vi "CTB4.vi"() -> ()   [LabVIEW 2015]
uses:
  <vilib>/Instr/_visa.llb/VISA Configure Serial Port (Instr).vi
  <vilib>/Utility/file.llb/Write Delimited Spreadsheet (I64).vi
panel:
  out "Mixed Signal Graph 2":T1(graph)
  in  "tiempo de muestreo":u32
  in  "timeout (10sec)":u32=10000
  in  "stop bits (10: 1 bit)":u16(ring)=10 items=["1.0"=10, "1.5"=15, "2.0"=20]
  in  "data bits (8)":u16=8 min=5 max=8 step=1
  in  "baud rate (9600)":u32=9600
  in  "VISA resource name 2":refnum<visa-resource-name>
  in  "Archivo":path
  out "?":u32[][](array[numeric])
  out "Muestras":i32
  in  "?":bool
  out "read buffer":string
  # "CH2"
  # "CH3"
  # "CH4"
  # "CH5"
  # "CH7"
  # "CH1"
  # "CH6"
  # "CH8"
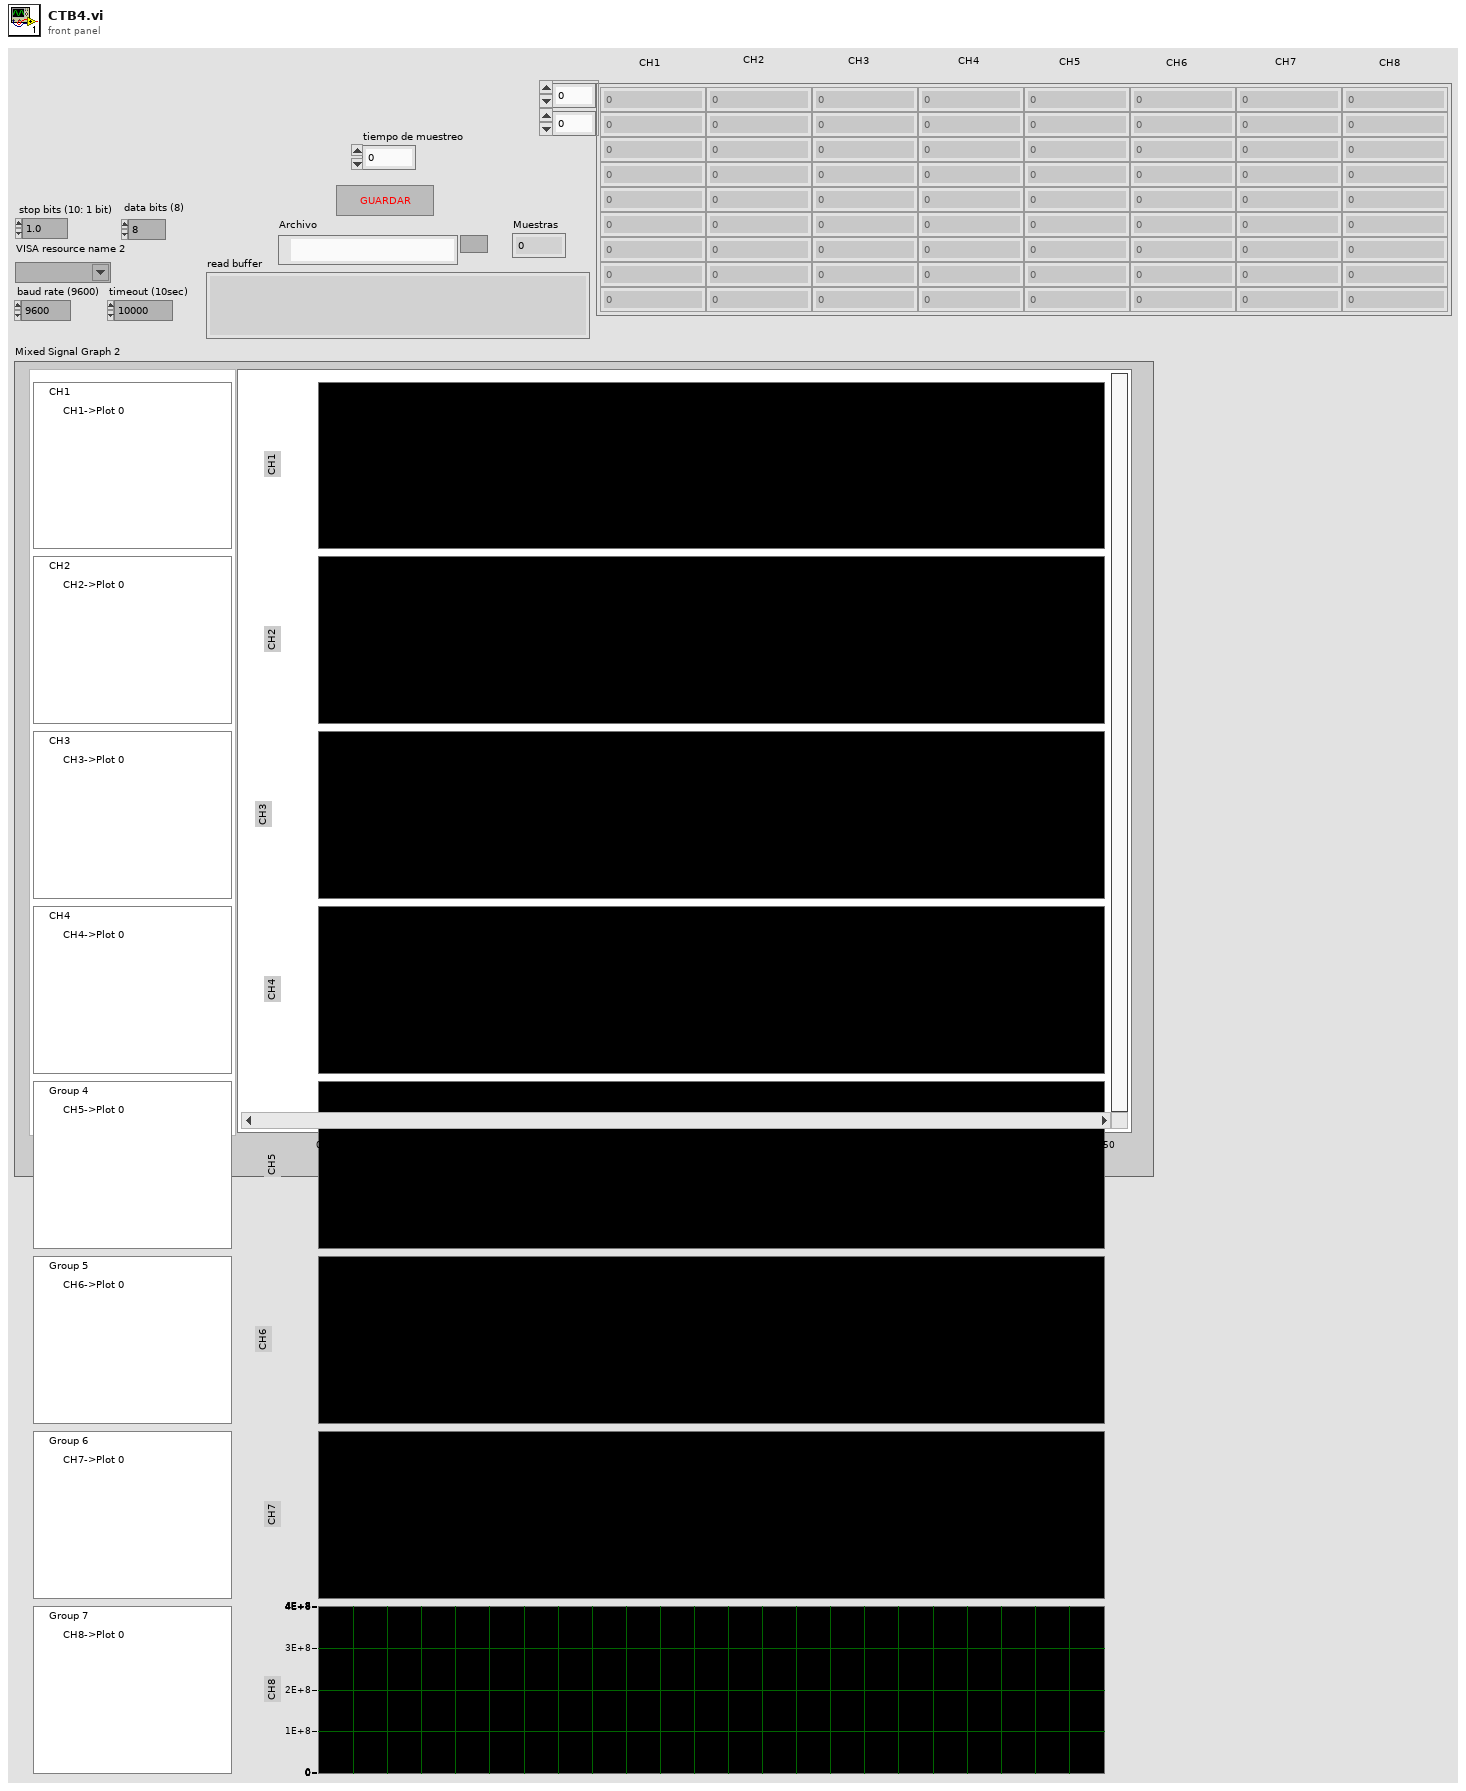
[diagram p1: front panel]
types:
  T1 = cluster{i32[], i32[], i32[], i32[], i32[], i32[], i32[], i32[]}
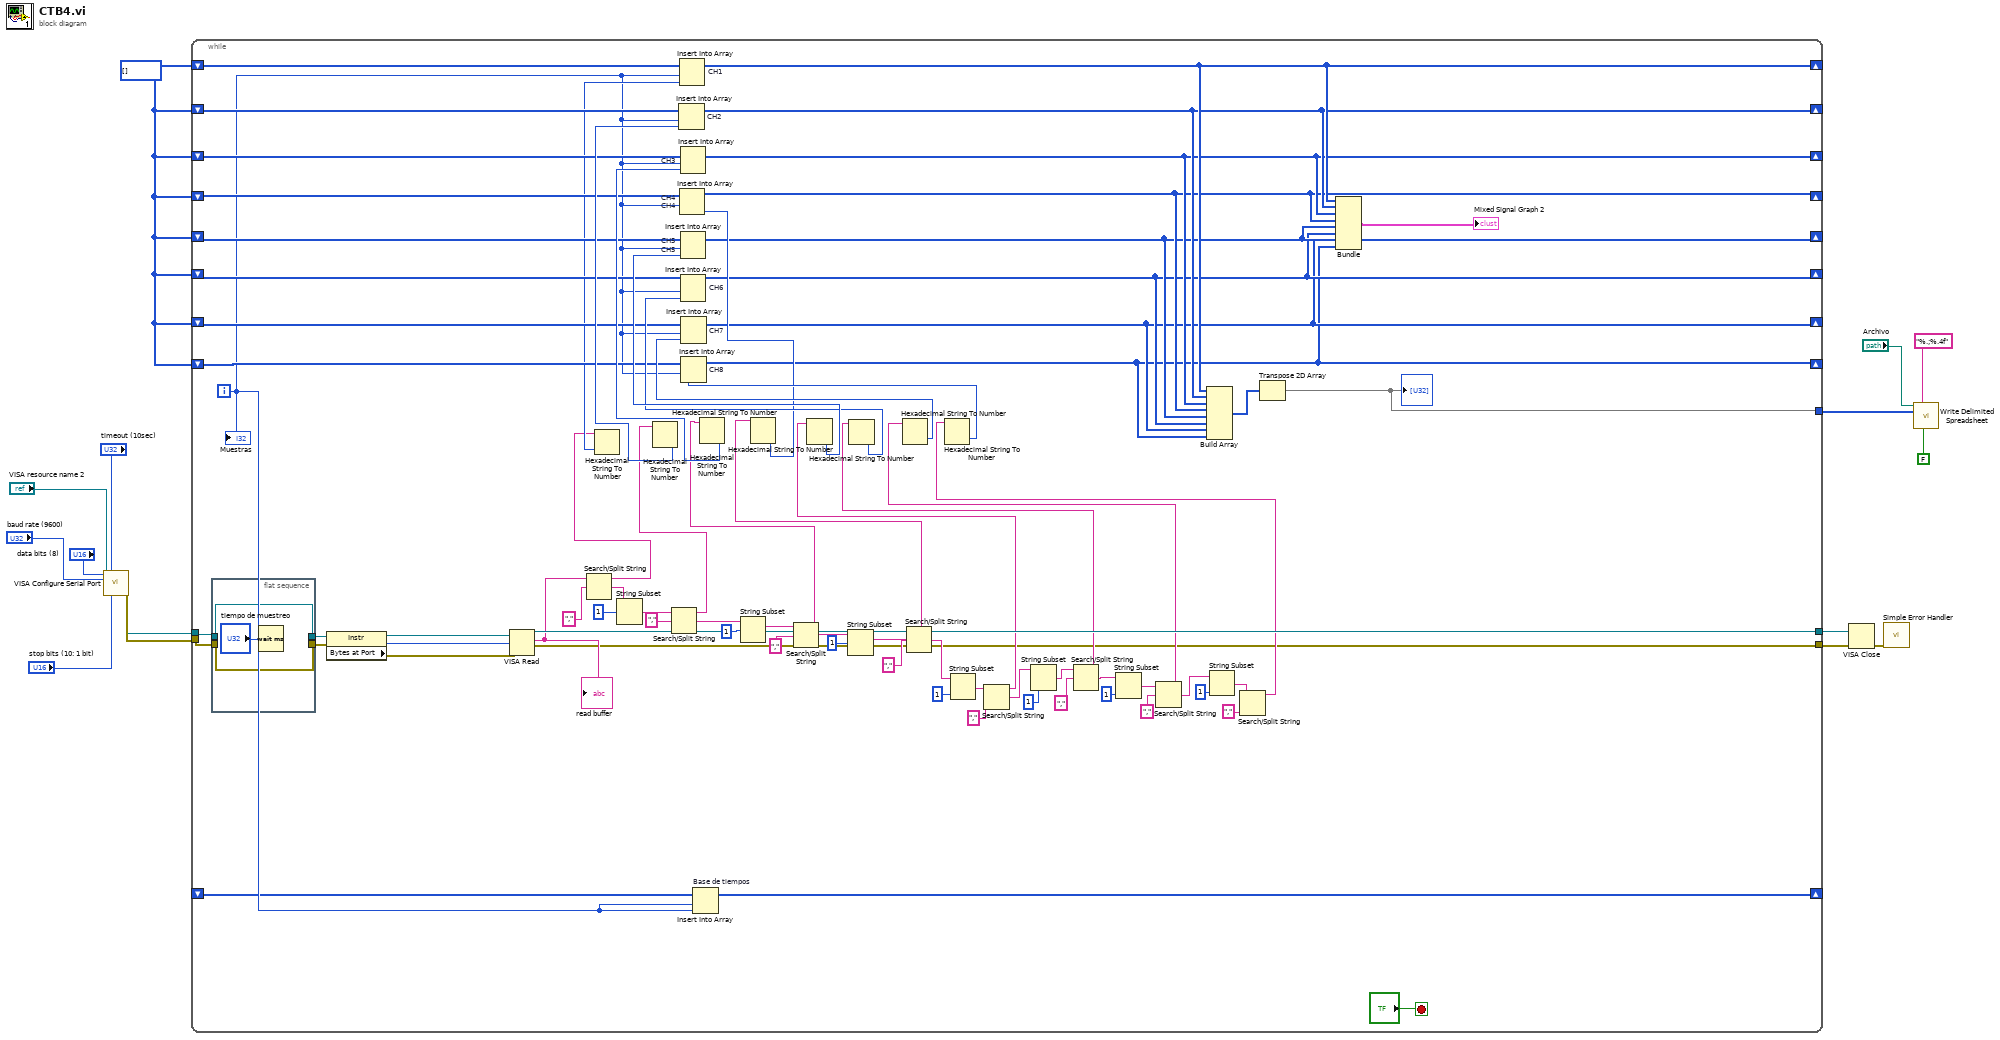
[diagram p0: block diagram]
diagram:
  w2 = i32[] []
  n1 = call-poly "VISA Configure Serial Port"("VISA resource name"="VISA resource name 2", "timeout (10sec)"="timeout (10sec)", "baud rate (9600)"="baud rate (9600)", "data bits (8)"="data bits (8)", "stop bits (10: 1 bit)"="stop bits (10: 1 bit)") -> ("VISA resource name out"=w5:refnum<visa-resource-name>, "error out"=w6:errorcluster)  [unwired: 9 in]
  n2 = while {
    shift-right: [w24] -> _
    shift-left: w2 -> [w33]
    shift-right: [w23] -> _
    shift-left: w2 -> [w86]
    shift-right: [w22] -> _
    shift-left: w2 -> [w83]
    shift-right: [w21] -> _
    shift-left: w2 -> [w78]
    shift-right: [w20] -> _
    shift-left: w2 -> [w77]
    shift-right: [w19] -> _
    shift-left: w2 -> [w67]
    shift-right: [w18] -> _
    shift-left: w2 -> [w66]
    shift-right: [w17] -> _
    shift-left: w2 -> [w65]
    tunnel: [w40] -> w13
    tunnel: w5 -> [w62]
    tunnel: w6 -> [w61]
    tunnel: [w64] -> w4
    shift-right: [w29] -> _
    shift-left: _ -> [w30]
    tunnel: [w27] -> w1
    i -> [w31]
    stop <- "?" stop-if-true
    n3 = flat-sequence {
      tunnel: w62 -> [w96]
      tunnel: [w96] -> w63
      tunnel: w61 -> [w95]
      tunnel: [w95] -> w60
      frame #0 {
        n4 = Wait (ms)(milliseconds to wait="tiempo de muestreo") -> ()  [unwired: 1 out]
      }
    }
    n5 = property class="Instr"(reference=w63, error in=w60) -> (reference out=w93:refnum<visa-resource-name>, error out=w28:errorcluster, "Bytes at Port"=w92:u32)
    n6 = VISA Read(VISA resource name=w93, byte count=w92, error in (no error)=w28) -> (VISA resource name out=w64:refnum<visa-resource-name>, read buffer=w32:string, error out=w27:errorcluster)  [unwired: 1 out]
    "read buffer" <- w32
    n7 = Search/Split String(string=w32, search string/char (-)=",") -> (substring before match=w26:string, match + rest of string=w89:string)  [unwired: 1 in, 1 out]
    n8 = Hexadecimal String To Number(string=w26) -> (number=w34:u32)  [unwired: 2 in, 1 out]
    n9 = String Subset(string=w89, offset (0)=1) -> (substring=w82:string)  [unwired: 1 in]
    n10 = Search/Split String(string=w82, search string/char (-)=",") -> (substring before match=w57:string, match + rest of string=w80:string)  [unwired: 1 in, 1 out]
    n11 = Hexadecimal String To Number(string=w57) -> (number=w87:u32)  [unwired: 2 in, 1 out]
    n12 = Insert Into Array "CH2"(array=w86, index=w31, new element=w87) -> (w23:i32[])
    n13 = Insert Into Array "CH1"(array=w33, index=w31, new element=w34) -> (w24:i32[])
    n14 = Insert Into Array "Base de tiempos"(array=w30, index=w31, new element=w31) -> (w29:i32[])
    n15 = String Subset(string=w80, offset (0)=1) -> (substring=w59:string)  [unwired: 1 in]
    n16 = Search/Split String(string=w59, search string/char (-)=",") -> (substring before match=w56:string, match + rest of string=w74:string)  [unwired: 1 in, 1 out]
    n17 = Hexadecimal String To Number(string=w56) -> (number=w84:u32)  [unwired: 2 in, 1 out]
    n18 = Insert Into Array "CH3"(array=w83, index=w31, new element=w84) -> (w22:i32[])
    n19 = String Subset(string=w74, offset (0)=1) -> (substring=w58:string)  [unwired: 1 in]
    n20 = Search/Split String(string=w58, search string/char (-)=",") -> (substring before match=w55:string, match + rest of string=w70:string)  [unwired: 1 in, 1 out]
    n21 = Hexadecimal String To Number(string=w55) -> (number=w35:u32)  [unwired: 2 in, 1 out]
    n22 = Insert Into Array "CH4\nCH4"(array=w78, index=w31, new element=w35) -> (w21:i32[])
    n23 = String Subset(string=w70, offset (0)=1) -> (substring=w53:string)  [unwired: 1 in]
    n24 = Search/Split String(string=w53, search string/char (-)=",") -> (substring before match=w39:string, match + rest of string=w49:string)  [unwired: 1 in, 1 out]
    n25 = Hexadecimal String To Number(string=w39) -> (number=w76:u32)  [unwired: 2 in, 1 out]
    n26 = Insert Into Array "CH5\nCH5"(array=w77, index=w31, new element=w76) -> (w20:i32[])
    n27 = String Subset(string=w49, offset (0)=1) -> (substring=w50:string)  [unwired: 1 in]
    n28 = Search/Split String(string=w50, search string/char (-)=",") -> (substring before match=w38:string, match + rest of string=w45:string)  [unwired: 1 in, 1 out]
    n29 = Hexadecimal String To Number(string=w38) -> (number=w68:u32)  [unwired: 2 in, 1 out]
    n30 = Insert Into Array "CH6"(array=w67, index=w31, new element=w68) -> (w19:i32[])
    n31 = String Subset(string=w45, offset (0)=1) -> (substring=w46:string)  [unwired: 1 in]
    n32 = Search/Split String(string=w46, search string/char (-)=",") -> (substring before match=w37:string, match + rest of string=w41:string)  [unwired: 1 in, 1 out]
    n33 = Hexadecimal String To Number(string=w37) -> (number=w72:u32)  [unwired: 2 in, 1 out]
    n34 = Insert Into Array "CH7"(array=w66, index=w31, new element=w72) -> (w18:i32[])
    n35 = String Subset(string=w41, offset (0)=1) -> (substring=w42:string)  [unwired: 1 in]
    n36 = Search/Split String(string=w42, search string/char (-)=",") -> (substring before match=w36:string)  [unwired: 1 in, 2 out]
    n37 = Hexadecimal String To Number(string=w36) -> (number=w69:u32)  [unwired: 2 in, 1 out]
    n38 = Insert Into Array "CH8"(array=w65, index=w31, new element=w69) -> (w17:i32[])
    n39 = Build Array "Build Array"(w24, w23, w22, w21, w20, w19, w18, w17) -> (w25:i32[][])
    n40 = Transpose 2D Array(2D array=w25) -> (transposed array=w40:i32[][])
    "?" <- w40
    n41 = Bundle(w24, w23, w22, w21, w20, w19, w18, w17) -> (→"Mixed Signal Graph 2":T1)  [unwired: 1 in]
    "Muestras" <- w31
  }
  n42 = VISA Close(VISA resource name=w4, error in (no error)=w1) -> (error out=w3:errorcluster)
  n43 = call <vilib>:"Simple Error Handler.vi"("error in (no error)"=w3) -> ()  [unwired: 4 in, 5 out]
  n44 = call-poly <vilib>:"Write Delimited Spreadsheet.vi"("file path (dialog if empty)"="Archivo", "format (%d)"="%.;%.4f" ("format (%.3f)"), "2D data"=w13, "transpose? (F)"=FALSE ("transpose? (no:F)")) -> ()  [unwired: 10 in, 2 out]
